vi "Update All Frame End Packet Frame IDs.vi"(0 "tagged llp packets cluster":T1, 1 "reset":bool, 9 "input valid":bool[](array[boolean])=[FALSE, FALSE, FALSE, FALSE, FALSE, FALSE, FALSE, FALSE], 12 "ready for output":bool[](array[boolean])=[FALSE, FALSE, FALSE, FALSE, FALSE, FALSE, FALSE, FALSE]) -> (4 "tagged llp packets cluster":T1, 10 "output valid":bool[](array[boolean]), 14 "ready for input":bool[](array[boolean]))   [LabVIEW 2020, in "GettingStarted_Common_148X_FPGA.lvlib"]
uses:
  GettingStarted_Common_148X_FPGA.lvlib
  Types/Tagged LLP Packets Cluster.ctl
  <instrlib>/FlexRIO/CSI-2/v2/FPGA/Types/Tagged LLP Packet.ctl
  <instrlib>/FlexRIO/CSI-2/v2/FPGA/Types/FPGA LLP Packet Tag.ctl
  <instrlib>/FlexRIO/CSI-2/v2/FPGA/Types/FPGA LLP Packet Timestamp.ctl
  <instrlib>/FlexRIO/CSI-2/v2/FPGA/Types/Timestamp ID.ctl
  <instrlib>/FlexRIO/CSI-2/v2/FPGA/Types/FPGA LLP Packet Size.ctl
  <instrlib>/FlexRIO/CSI-2/v2/FPGA/Types/LLP Packet.ctl
  <instrlib>/FlexRIO/CSI-2/v2/FPGA/Types/LLP Packet Header.ctl
  <instrlib>/FlexRIO/CSI-2/v2/FPGA/Types/LLP Packet Payload.ctl
  <instrlib>/FlexRIO/CSI-2/v2/FPGA/Types/LLP Packet Footer.ctl
  <instrlib>/_niInstr/Basic Elements/v1/FPGA/niInstr Basic Elements v1 FPGA.lvlib
  <instrlib>/FlexRIO/CSI-2/v2/FPGA/NI CSI-2 API FPGA v2.lvlib
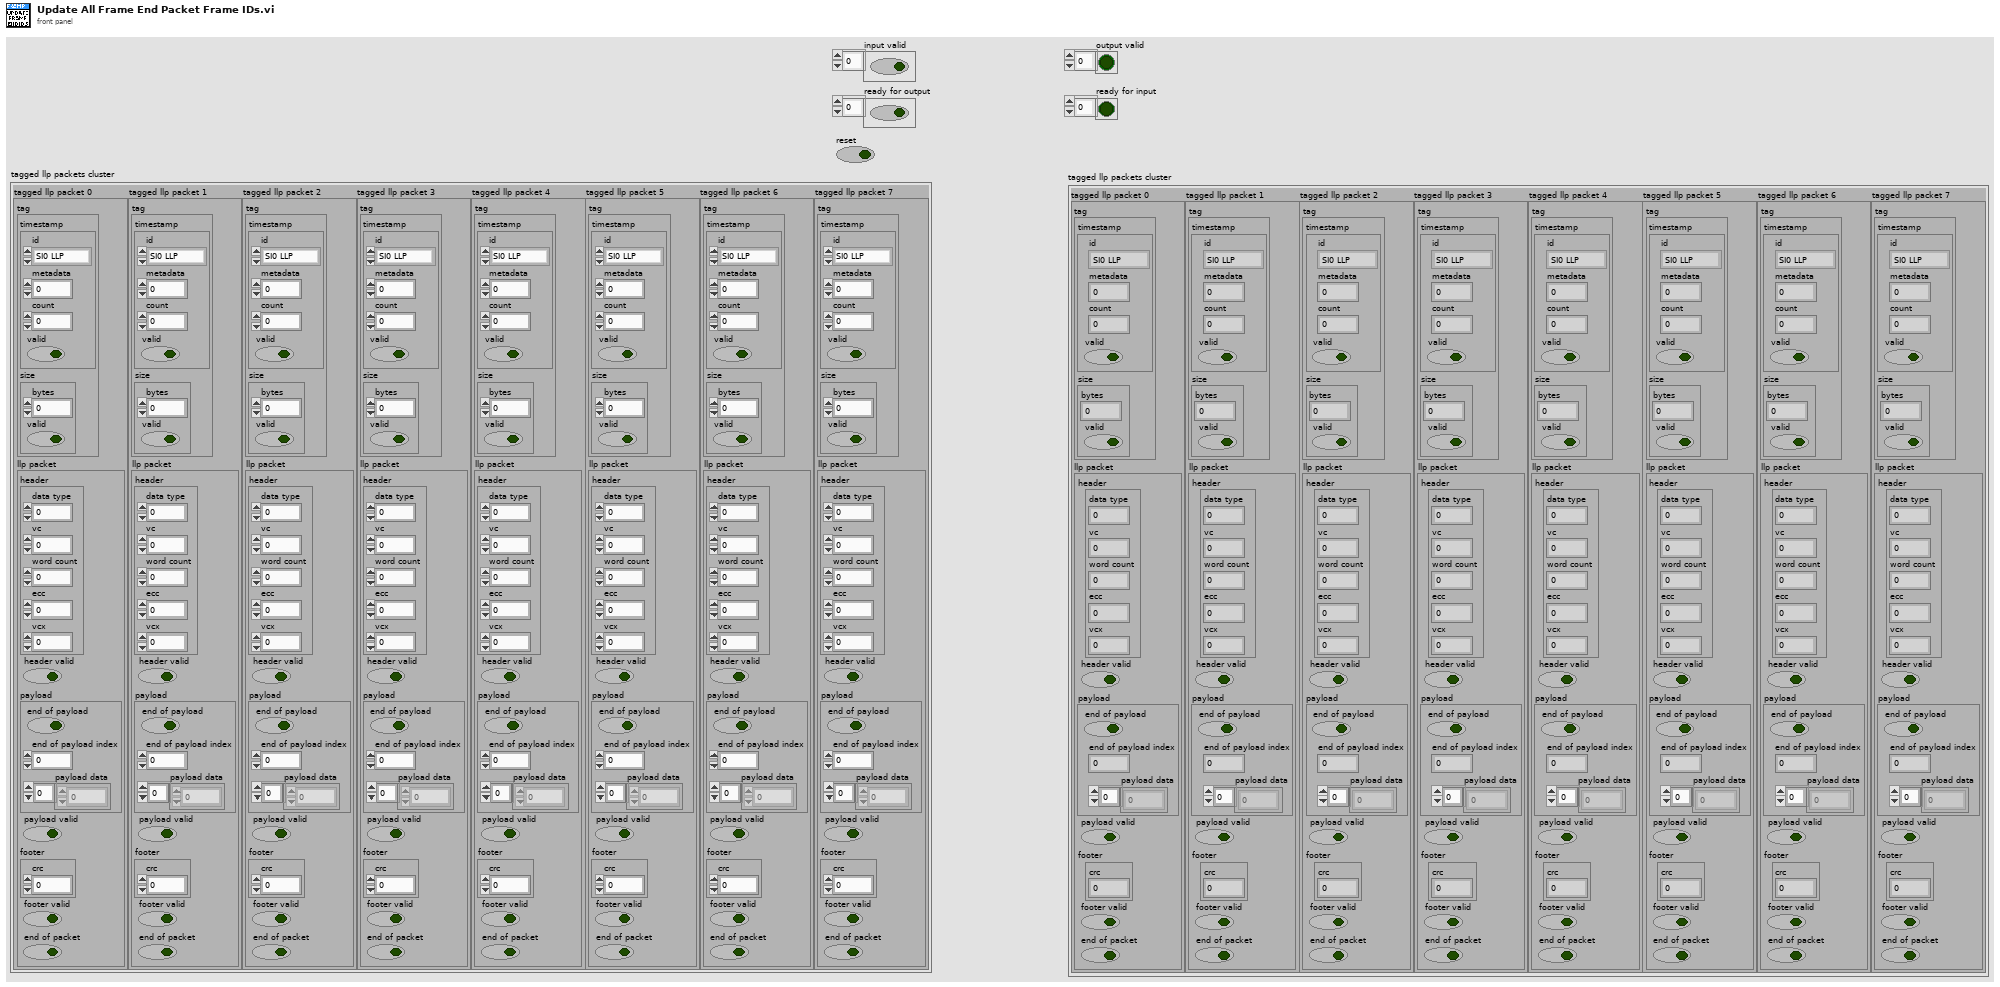
[diagram p1: front panel]
types:
  T1 = typedef "GettingStarted_Common_148X_FPGA.lvlib/Tagged LLP Packets Cluster.ctl" = cluster{"tagged llp packet 0":T2, "tagged llp packet 1":T2, "tagged llp packet 2":T2, "tagged llp packet 3":T2, "tagged llp packet 4":T2, "tagged llp packet 5":T2, "tagged llp packet 6":T2, "tagged llp packet 7":T2}
  T2 = typedef "NI CSI-2 API FPGA v2.lvlib/Tagged LLP Packet.ctl" = cluster{"tag":T3, "llp packet":T7}
  T3 = typedef "NI CSI-2 API FPGA v2.lvlib/FPGA LLP Packet Tag.ctl" = cluster{"timestamp":T4, "size":T6}
  T4 = typedef "NI CSI-2 API FPGA v2.lvlib/FPGA LLP Packet Timestamp.ctl" = cluster{"valid":bool, "count":fxp<+,50,50>, "id":T5, "metadata":u8}
  T5 = typedef "NI CSI-2 API FPGA v2.lvlib/Timestamp ID.ctl" = enum8{"SI0 LLP", "SI1 LLP", "SI2 LLP", "SI3 LLP", "SI4 LLP", "SI5 LLP", "SI6 LLP", "SI7 LLP", "SO0 LLP", "SO1 LLP", "SO2 LLP", "SO3 LLP", "SO4 LLP", "SO5 LLP", "SO6 LLP", "SO7 LLP", "Ser0 GPIO Bank", "Ser1 GPIO Bank", "Ser2 GPIO Bank", "Ser3 GPIO Bank", "Ser4 GPIO Bank", "Ser5 GPIO Bank", "Ser6 GPIO Bank", "Ser7 GPIO Bank", "Des0 GPIO Bank", "Des1 GPIO Bank", "Des2 GPIO Bank", "Des3 GPIO Bank", "Des4 GPIO Bank", "Des5 GPIO Bank", "Des6 GPIO Bank", "Des7 GPIO Bank", "User0", "User1", "User2", "User3", "User4", "User5", "User6", "User7", "User8", "User9", "User10", "User11", "User12", "User13", "User14", "User15", "User16", "User17", "User18", "User19", "User20", "User21", "User22", "User23", "User24", "User25", "User26", "User27", "User28", "User29", "User30", "User31"}
  T6 = typedef "NI CSI-2 API FPGA v2.lvlib/FPGA LLP Packet Size.ctl" = cluster{"bytes":fxp<+,17,17>, "valid":bool}
  T7 = typedef "NI CSI-2 API FPGA v2.lvlib/LLP Packet.ctl" = cluster{"header":T8, "header valid":bool, "payload":T9, "payload valid":bool, "footer":T10, "footer valid":bool, "end of packet":bool}
  T8 = typedef "NI CSI-2 API FPGA v2.lvlib/LLP Packet Header.ctl" = cluster{"word count":u16, "ecc":fxp<+,6,6>, "vcx":fxp<+,2,2>, "data type":fxp<+,6,6>, "vc":fxp<+,2,2>}
  T9 = typedef "NI CSI-2 API FPGA v2.lvlib/LLP Packet Payload.ctl" = cluster{"end of payload":bool, "end of payload index":fxp<+,3,3>, "payload data":u8[]}
  T10 = typedef "NI CSI-2 API FPGA v2.lvlib/LLP Packet Footer.ctl" = cluster{"crc":u16}
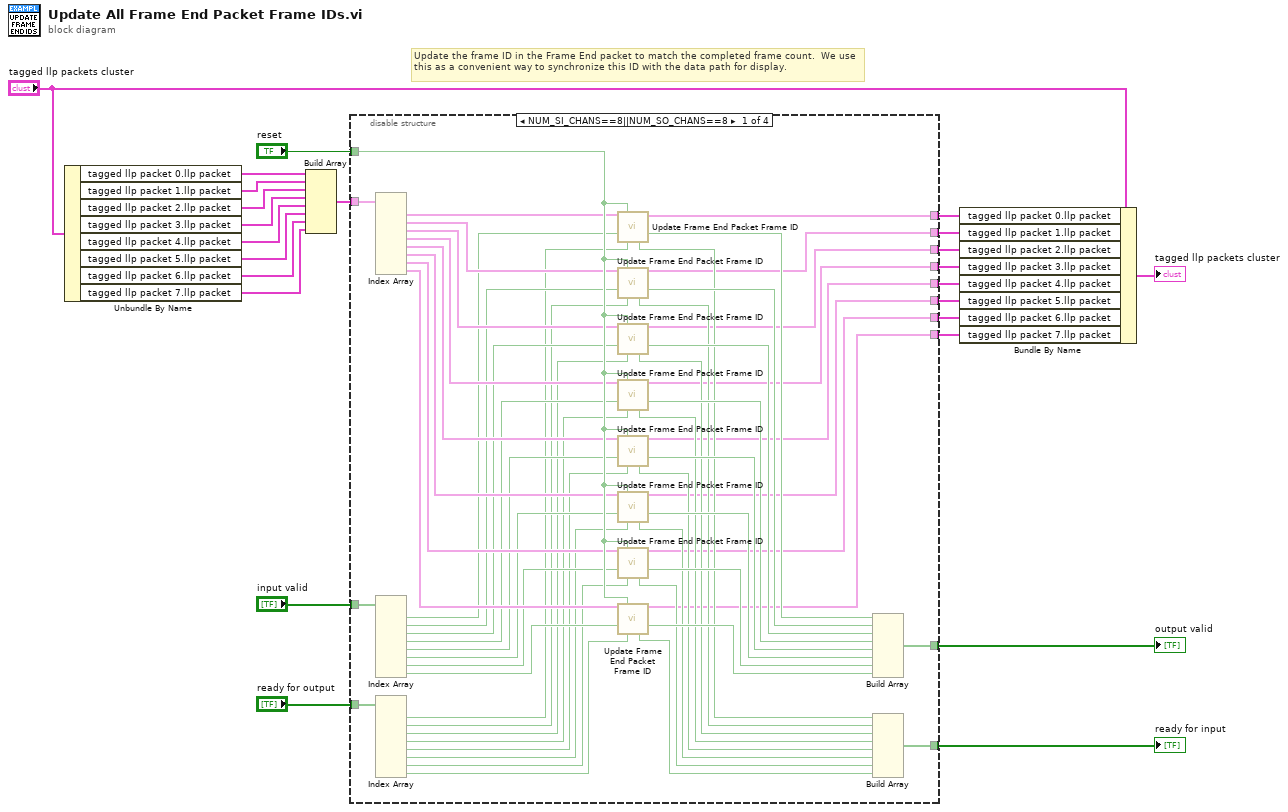
[diagram p0: block diagram]
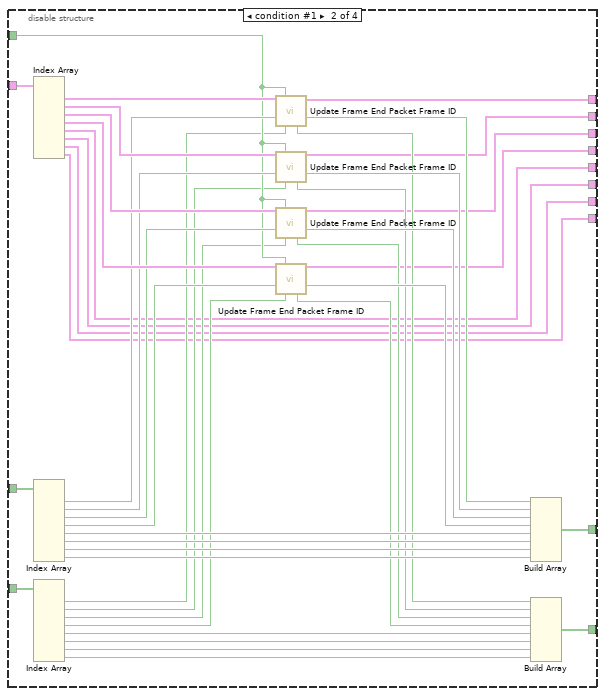
[diagram p2: hidden frame]
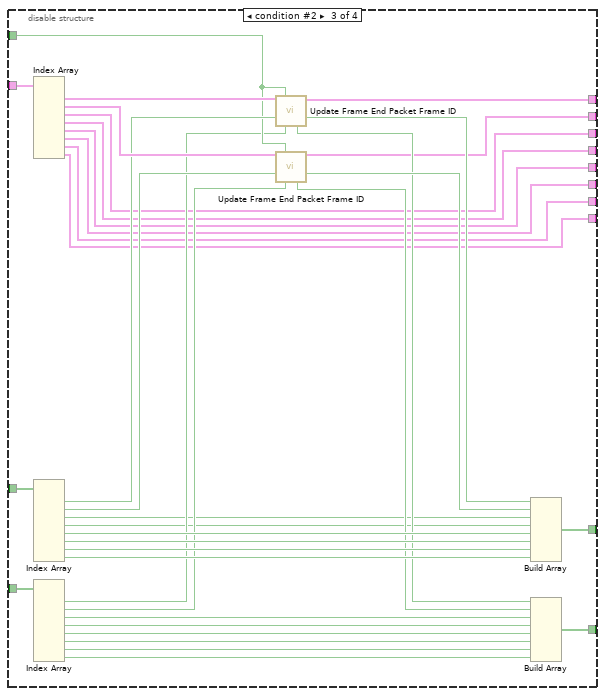
[diagram p3: hidden frame]
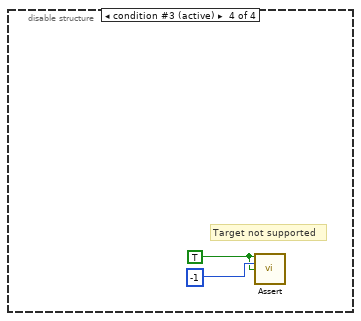
[diagram p4: hidden frame]
diagram:
  # "Update the frame ID in the Frame End packet to match the completed frame count.  We use this as a convenient way to synchronize this ID with the data path for display."
  n1 = Unbundle By Name("tagged llp packets cluster") -> ("tagged llp packet 0.llp packet"=w19:T7, "tagged llp packet 1.llp packet"=w18:T7, "tagged llp packet 2.llp packet"=w12:T7, "tagged llp packet 3.llp packet"=w13:T7, "tagged llp packet 4.llp packet"=w14:T7, "tagged llp packet 5.llp packet"=w15:T7, "tagged llp packet 6.llp packet"=w16:T7, "tagged llp packet 7.llp packet"=w17:T7)
  n2 = Build Array(w19, w18, w12, w13, w14, w15, w16, w17) -> (w11:T7[])
  n3 = disable-structure shown="NUM_SI_CHANS==8||NUM_SO_CHANS==8" {
    disable-tunnel: w11 -> [w78 w108 w150 _]
    disable-tunnel: "reset" -> [w77 w106 w148 _]
    disable-tunnel: "input valid" -> [w68 w107 w149 _]
    disable-tunnel: [w52 w101 w143 _] -> w22
    disable-tunnel: "ready for output" -> [w50 w100 w142 _]
    disable-tunnel: [w34 w99 w141 _] -> w20
    disable-tunnel: [w32 w79 w127 _] -> w9
    disable-tunnel: [w31 w80 w128 _] -> w8
    disable-tunnel: [w30 w81 w129 _] -> w7
    disable-tunnel: [w29 w82 w130 _] -> w6
    disable-tunnel: [w28 w83 w122 _] -> w5
    disable-tunnel: [w27 w84 w121 _] -> w4
    disable-tunnel: [w26 w85 w131 _] -> w3
    disable-tunnel: [w25 w86 w132 _] -> w2
    frame condition #0 {
      n4 = Index Array(array=w78) -> (element #1=w33:T7, element #2=w76:T7, element #3=w75:T7, element #4=w74:T7, element #5=w73:T7, element #6=w72:T7, element #7=w71:T7, element #8=w70:T7)  [unwired: 8 in]
      n5 = Index Array(array=w68) -> (element #1=w61:bool, element #2=w62:bool, element #3=w63:bool, element #4=w64:bool, element #5=w65:bool, element #6=w66:bool, element #7=w67:bool, element #8=w69:bool)  [unwired: 8 in]
      n6 = Index Array(array=w50) -> (element #1=w51:bool, element #2=w49:bool, element #3=w48:bool, element #4=w47:bool, element #5=w46:bool, element #6=w45:bool, element #7=w44:bool, element #8=w43:bool)  [unwired: 8 in]
      n7 = call "Update Frame End Packet Frame ID.vi"("llp packet in"=w33, "reset"=w77, "input valid"=w61, "ready for output"=w51) -> ("llp packet out"=w25:T7, "output valid"=w60:bool, "ready for input"=w42:bool)  [unwired: 9 in]
      n8 = call "Update Frame End Packet Frame ID.vi"("llp packet in"=w76, "reset"=w77, "input valid"=w62, "ready for output"=w49) -> ("llp packet out"=w26:T7, "output valid"=w59:bool, "ready for input"=w41:bool)  [unwired: 9 in]
      n9 = call "Update Frame End Packet Frame ID.vi"("llp packet in"=w75, "reset"=w77, "input valid"=w63, "ready for output"=w48) -> ("llp packet out"=w27:T7, "output valid"=w58:bool, "ready for input"=w40:bool)  [unwired: 9 in]
      n10 = call "Update Frame End Packet Frame ID.vi"("llp packet in"=w74, "reset"=w77, "input valid"=w64, "ready for output"=w47) -> ("llp packet out"=w28:T7, "output valid"=w57:bool, "ready for input"=w39:bool)  [unwired: 9 in]
      n11 = call "Update Frame End Packet Frame ID.vi"("llp packet in"=w73, "reset"=w77, "input valid"=w65, "ready for output"=w46) -> ("llp packet out"=w29:T7, "output valid"=w56:bool, "ready for input"=w38:bool)  [unwired: 9 in]
      n12 = call "Update Frame End Packet Frame ID.vi"("llp packet in"=w72, "reset"=w77, "input valid"=w66, "ready for output"=w45) -> ("llp packet out"=w30:T7, "output valid"=w55:bool, "ready for input"=w37:bool)  [unwired: 9 in]
      n13 = call "Update Frame End Packet Frame ID.vi"("llp packet in"=w71, "reset"=w77, "input valid"=w67, "ready for output"=w44) -> ("llp packet out"=w31:T7, "output valid"=w54:bool, "ready for input"=w36:bool)  [unwired: 9 in]
      n14 = call "Update Frame End Packet Frame ID.vi"("llp packet in"=w70, "reset"=w77, "input valid"=w69, "ready for output"=w43) -> ("llp packet out"=w32:T7, "output valid"=w53:bool, "ready for input"=w35:bool)  [unwired: 9 in]
      n15 = Build Array(w60, w59, w58, w57, w56, w55, w54, w53) -> (w52:bool[])
      n16 = Build Array(w42, w41, w40, w39, w38, w37, w36, w35) -> (w34:bool[])
    }
    frame condition #1 {
      n17 = Index Array(array=w108) -> (element #1=w120:T7, element #2=w119:T7, element #3=w118:T7, element #4=w117:T7, element #5=w82:T7, element #6=w81:T7, element #7=w80:T7, element #8=w79:T7)  [unwired: 8 in]
      n18 = Index Array(array=w107) -> (element #1=w113:bool, element #2=w114:bool, element #3=w115:bool, element #4=w116:bool, element #5=w102:bool, element #6=w103:bool, element #7=w104:bool, element #8=w105:bool)  [unwired: 8 in]
      n19 = Index Array(array=w100) -> (element #1=w90:bool, element #2=w89:bool, element #3=w88:bool, element #4=w87:bool, element #5=w91:bool, element #6=w92:bool, element #7=w93:bool, element #8=w94:bool)  [unwired: 8 in]
      n20 = call "Update Frame End Packet Frame ID.vi"("llp packet in"=w120, "reset"=w106, "input valid"=w113, "ready for output"=w90) -> ("llp packet out"=w86:T7, "output valid"=w112:bool, "ready for input"=w98:bool)  [unwired: 9 in]
      n21 = call "Update Frame End Packet Frame ID.vi"("llp packet in"=w119, "reset"=w106, "input valid"=w114, "ready for output"=w89) -> ("llp packet out"=w85:T7, "output valid"=w111:bool, "ready for input"=w97:bool)  [unwired: 9 in]
      n22 = call "Update Frame End Packet Frame ID.vi"("llp packet in"=w118, "reset"=w106, "input valid"=w115, "ready for output"=w88) -> ("llp packet out"=w84:T7, "output valid"=w110:bool, "ready for input"=w96:bool)  [unwired: 9 in]
      n23 = call "Update Frame End Packet Frame ID.vi"("llp packet in"=w117, "reset"=w106, "input valid"=w116, "ready for output"=w87) -> ("llp packet out"=w83:T7, "output valid"=w109:bool, "ready for input"=w95:bool)  [unwired: 9 in]
      n24 = Build Array(w112, w111, w110, w109, w102, w103, w104, w105) -> (w101:bool[])
      n25 = Build Array(w98, w97, w96, w95, w91, w92, w93, w94) -> (w99:bool[])
    }
    frame condition #2 {
      n26 = Index Array(array=w150) -> (element #1=w156:T7, element #2=w155:T7, element #3=w121:T7, element #4=w122:T7, element #5=w130:T7, element #6=w129:T7, element #7=w128:T7, element #8=w127:T7)  [unwired: 8 in]
      n27 = Index Array(array=w149) -> (element #1=w153:bool, element #2=w154:bool, element #3=w125:bool, element #4=w126:bool, element #5=w144:bool, element #6=w145:bool, element #7=w146:bool, element #8=w147:bool)  [unwired: 8 in]
      n28 = Index Array(array=w142) -> (element #1=w134:bool, element #2=w133:bool, element #3=w124:bool, element #4=w123:bool, element #5=w135:bool, element #6=w136:bool, element #7=w137:bool, element #8=w138:bool)  [unwired: 8 in]
      n29 = call "Update Frame End Packet Frame ID.vi"("llp packet in"=w156, "reset"=w148, "input valid"=w153, "ready for output"=w134) -> ("llp packet out"=w132:T7, "output valid"=w152:bool, "ready for input"=w140:bool)  [unwired: 9 in]
      n30 = call "Update Frame End Packet Frame ID.vi"("llp packet in"=w155, "reset"=w148, "input valid"=w154, "ready for output"=w133) -> ("llp packet out"=w131:T7, "output valid"=w151:bool, "ready for input"=w139:bool)  [unwired: 9 in]
      n31 = Build Array(w152, w151, w125, w126, w144, w145, w146, w147) -> (w143:bool[])
      n32 = Build Array(w140, w139, w124, w123, w135, w136, w137, w138) -> (w141:bool[])
    }
    frame condition #3 (active) {
      w157 = TRUE ("assert")
      # "Target not supported"
      n33 = call <instrlib>:"Assert.vi"("assert"=w157, "error code"=-1, "enable show error"=w157) -> ()  [unwired: 13 in]
    }
  }
  "output valid" <- w22
  "ready for input" <- w20
  n34 = Bundle By Name(cluster="tagged llp packets cluster", "tagged llp packet 0.llp packet"=w2, "tagged llp packet 1.llp packet"=w3, "tagged llp packet 2.llp packet"=w4, "tagged llp packet 3.llp packet"=w5, "tagged llp packet 4.llp packet"=w6, "tagged llp packet 5.llp packet"=w7, "tagged llp packet 6.llp packet"=w8, "tagged llp packet 7.llp packet"=w9) -> (→"tagged llp packets cluster":T1)
